vi "DELAY-Completo.vi"(6 "error in (no error)":errorcluster, 8 "Byte4(0)":string, 9 "Byte3(0)":string, 10 "Byte2 (0)":string, 11 "Byte1 (0)":string) -> (0 "error out":errorcluster, 3 "DelayOut":string)   [LabVIEW 2014, in "CAP-USB.lvlib"]
doc: "Arma el comando correspondiente\npara implementar un delay en el CAP-USB.\nEl tiempo de delay se especifica en uS.\nLos valores de Byte 1 a 4 son el equivalente en \nASCII del valor en I32(decimal)"
uses:
  CAP-USB.lvlib
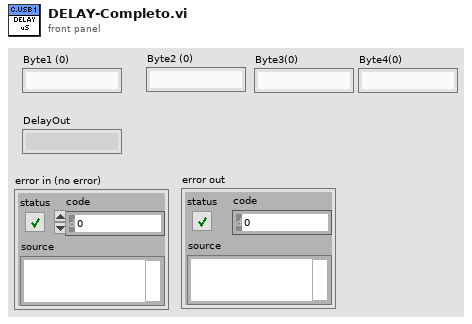
[diagram p1: front panel]
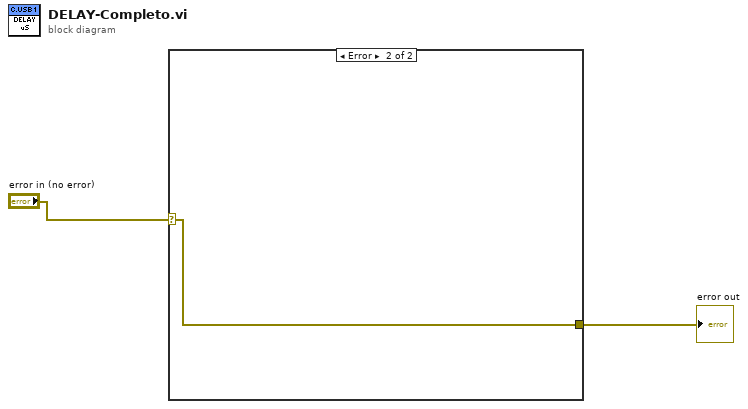
[diagram p0: block diagram]
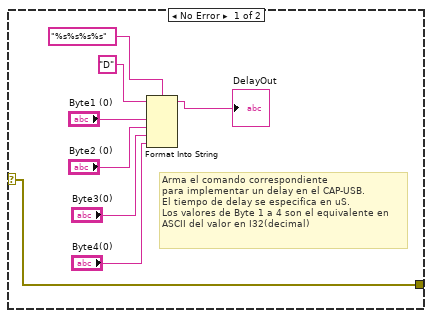
[diagram p2: hidden frame]
diagram:
  n1 = case shown="Error" "error in (no error)" {
    selector: "error in (no error)" -> [w3 w11]
    tunnel: [w3 w11] -> w1
    frame No Error {
      # "Arma el comando correspondiente\npara implementar un delay en el CAP-USB.\nEl tiempo de delay se especifica en uS.\nLos valores de Byte 1 a 4 son el equivalente en \nASCII del valor en I32(decimal)"
      n2 = Format Into String(format string="%s%s%s%s", initial string="D" ("DELAY(D)"), "Byte1 (0)", "Byte2 (0)", "Byte3(0)", "Byte4(0)") -> (resulting string=→"DelayOut":string)  [unwired: 1 in, 1 out]
    }
    frame Error {
    }
  }
  "error out" <- w1
